vi "niRFUtil CONV dBm to 1 Ohm Watt (real wfm).vi"(7 "Real Waveform (dBm)":T1 {"y" min=0 max=127 format="%.2f"; "dx" format="%^.2e"; "x0" format="%^.2e"}) -> (8 "Real Waveform (W)":T1 {"y" min=0 max=127 format="%.2f"; "dx" format="%^.2e"; "x0" format="%^.2e"})   [LabVIEW 2015, in "niRFUtil.lvlib"]
doc: "(c) Copyright 2006, National Instruments, Inc. This VI may not be duplicated, sold, or distributed without written consent from National Instruments."
uses:
  niRFUtil.lvlib
  Includes/niRFUtil INC Real Waveform.ctl
  Includes/niRFUtil INC Real Array.ctl
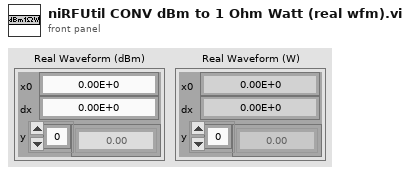
[diagram p1: front panel]
types:
  T1 = typedef "niRFUtil.lvlib/niRFUtil INC Real Waveform.ctl" = cluster{"x0":dbl, "dx":dbl, "y":T2}
  T2 = typedef "niRFUtil.lvlib/niRFUtil INC Real Array.ctl" = sgl[]
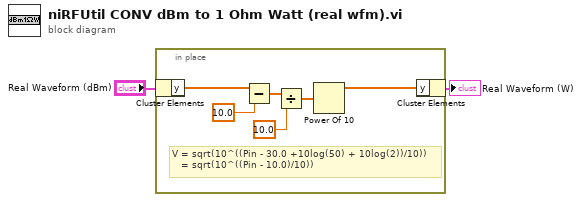
[diagram p0: block diagram]
diagram:
  n1 = in-place {
    # "V = sqrt(10^((Pin - 30.0 +10log(50) + 10log(2))/10))\n   = sqrt(10^((Pin - 10.0)/10))"
    n2 = in-place-cluster #1("Real Waveform (dBm)") -> ("y"=w4:T2)
    n3 = Subtract(x=w4, y=sgl 10.0) -> (x-y=w8:T2)
    n4 = Divide(x=w8, y=sgl 10.0) -> (x/y=w6:T2)
    n5 = Power Of 10(x=w6) -> (10^x=w3:T2)
    n6 = in-place-cluster #1("y"=w3) -> (→"Real Waveform (W)":T1)
  }
